vi "Update-splitter-references.vi"(8 "error in (no error)":errorcluster, 10 "Sorted splitter references":refnum<vi>[](array[refnum]), 11 "Pane in":T1) -> (0 "error out":errorcluster, 3 "Pane out":T1)   [LabVIEW 2013, in "CameraVision.lvlib" / "CV-Panes.lvclass"]
uses:
  CV-Panes.lvclass
  Pane-settings.ctl
  Pane-names.ctl
  Splitter-settings.ctl
  Splitter-names.ctl
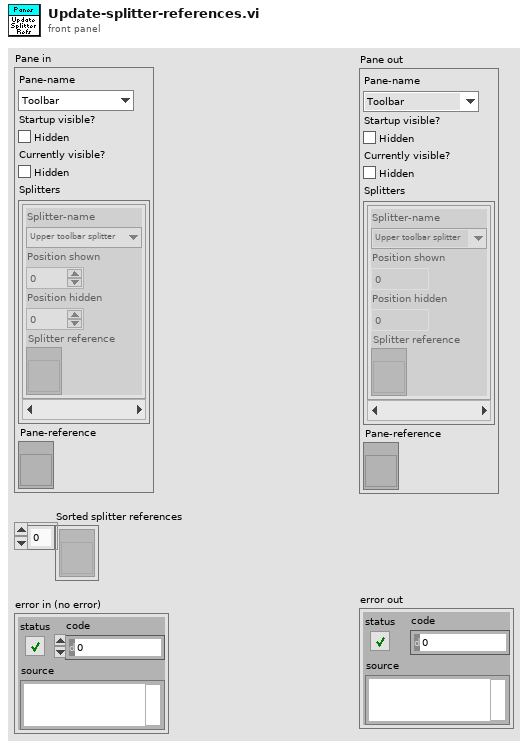
[diagram p1: front panel]
types:
  T1 = typedef "CameraVision.lvlib/CV-Panes.lvclass/Pane-settings.ctl" = cluster{"Pane-name":T2, "Startup visible?":bool, "Currently visible?":bool, "Splitters":T3[], "Pane-reference":refnum<vi>}
  T2 = typedef "CameraVision.lvlib/CV-Panes.lvclass/Pane-names.ctl" = enum16{"Toolbar", "Help bar", "Toolbar lower border", "Settings", "Displays", "Status bar upper border", "General state bar", "Information bar"}
  T3 = typedef "CameraVision.lvlib/CV-Panes.lvclass/Splitter-settings.ctl" = cluster{"Splitter-name":T4, "Position shown":i32, "Position hidden":i32, "Splitter reference":refnum<vi>}
  T4 = typedef "CameraVision.lvlib/CV-Panes.lvclass/Splitter-names.ctl" = enum16{"Upper toolbar splitter", "Help bar splitter", "Lower toolbar splitter", "Upper status bar splitter", "Lower status bar splitter", "Splitter", "Settings splitter"}
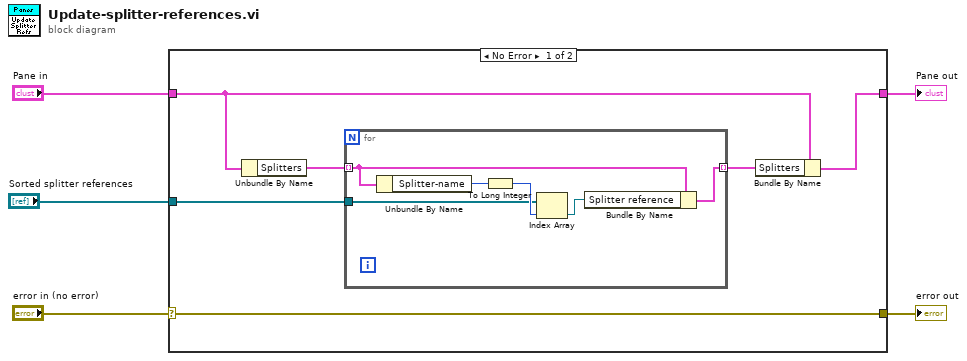
[diagram p0: block diagram]
diagram:
  n1 = case shown="No Error" "error in (no error)" {
    selector: "error in (no error)" -> [w7 w18]
    tunnel: [w11 w19] -> w5
    tunnel: "Pane in" -> [w9 w19]
    tunnel: "Sorted splitter references" -> [w8 _]
    tunnel: [w7 w18] -> w1
    frame No Error {
      n2 = Unbundle By Name(w9) -> ("Splitters"=w6:T3[])
      n3 = for {
        tunnel: [w12] -> w10 mode=indexing
        tunnel: w8 -> [w16]
        tunnel: w6 -> [w13] mode=indexing
        n4 = Unbundle By Name(w13) -> ("Splitter-name"=w15:T4)
        n5 = To Long Integer(number=w15) -> (32bit integer=w17:i32)
        n6 = Index Array(array=w16, index=w17) -> (element=w14:refnum<vi>)
        n7 = Bundle By Name(cluster=w13, "Splitter reference"=w14) -> (w12:T3)
      }
      n8 = Bundle By Name(cluster=w9, "Splitters"=w10) -> (w11:T1)
    }
    frame Error {
    }
  }
  "error out" <- w1
  "Pane out" <- w5
